vi "F Moments.vi"(9 "k2":i32=1, 10 "k1":i32=1) -> (0 "error":i32, 2 "variance":dbl=1.0, 3 "mean":dbl)   [LabVIEW 2014, in "NI_Gmath.lvlib"]
doc: "Returns the expected mean and variance of the random variate X, where X describes the selected distribution type. You must manually select the polymorphic instance to use."
uses:
  NI_Gmath.lvlib
  st_error_code.ctl
panel:
  # "F Moments"
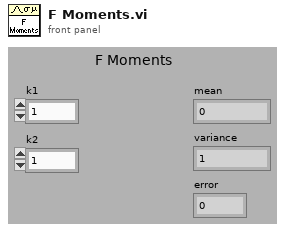
[diagram p1: front panel]
types:
  T1 = typedef "NI_Gmath.lvlib/st_error_code.ctl" = i32
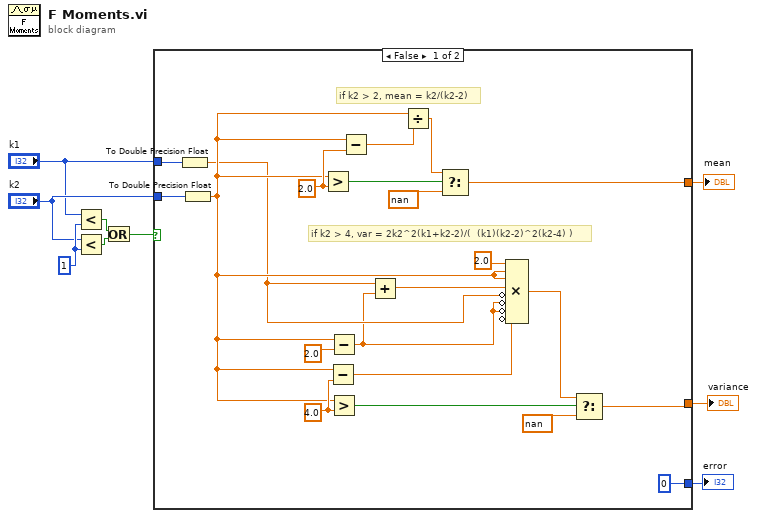
[diagram p0: block diagram]
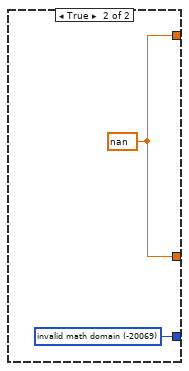
[diagram p2: hidden frame]
diagram:
  w4 = 1 ("y")
  n1 = Less?(x="k1", y=w4) -> (x < y?=w5:bool)
  n2 = Less?(x="k2", y=w4) -> (x < y?=w6:bool)
  n3 = Or(x=w5, y=w6) -> (x .or. y?=w7:bool)
  n4 = case shown="False" w7 {
    tunnel: "k2" -> [w25 _]
    tunnel: [0 ("invalid math domain") w31] -> w9
    tunnel: [w23 w32] -> w8
    tunnel: "k1" -> [w29 _]
    tunnel: [w16 w32] -> w1
    frame False {
      w18 = 4.0 ("k2")
      w19 = 2.0 ("k2")
      # "if k2 > 4, var = 2k2^2(k1+k2-2)/(  (k1)(k2-2)^2(k2-4) )"
      # "if k2 > 2, mean = k2/(k2-2)"
      n5 = To Double Precision Float(number=w29) -> (double precision float=w12:dbl)
      n6 = To Double Precision Float(number=w25) -> (double precision float=w14:dbl)
      n7 = Greater?(x=w14, y=w19) -> (0:w27:bool)
      n8 = Subtract(x=w14, y=w18) -> (x-y=w15:dbl)
      n9 = Subtract(x=w14, y=2.0 ("k2")) -> (x-y=w11:dbl)
      n10 = Greater?(x=w14, y=w18) -> (0:w22:bool)
      n11 = Subtract(x=w14, y=w19) -> (x-y=w26:dbl)
      n12 = Add(x=w12, y=w11) -> (x+y=w10:dbl)
      n13 = Divide(x=w14, y=w26) -> (x/y=w24:dbl)
      n14 = Select(t=w24, s=w27, f=nan) -> (s? t:f=w23:dbl)
      n15 = Compound Arithmetic op=MULTIPLY(2.0 ("k2"), w14, w14, w10, invert w12, invert w11, invert w11, invert w15) -> (w17:dbl)
      n16 = Select(t=w17, s=w22, f=nan) -> (s? t:f=w16:dbl)
    }
    frame True {
      w31 = T1 -20069 items=["invalid math domain"=-20069, "Fourier interpolation size m >= n"=-20070, "empty array"=-20003] ("stat interp error code")
      w32 = nan
    }
  }
  "mean" <- w8
  "error" <- w9
  "variance" <- w1
